vi "test-telemetry_engine.vi"() -> ()   [LabVIEW 2017, in "labview-standard-library.lvlib" / "data-logging.lvlib"]
uses:
  data-logging.lvlib
  <vilib>/Rock Robotics/WPI/DriverStation/WPI_DriverStationRobotMode2.ctl
panel:
  in  "Post dissable record time":dbl=10.0 format="%#_13g"
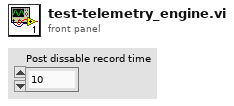
[diagram p1: front panel]
types:
  T1 = typedef "WPI_DriverStationRobotMode2.ctl" = enum16{"Autonomous Disabled", "Autonomous Enabled", "Teleop Disabled", "Teleop Enabled", "Disconnected", "Finish", "Test Disabled", "Test Enabled", "Emergency Stopped"}
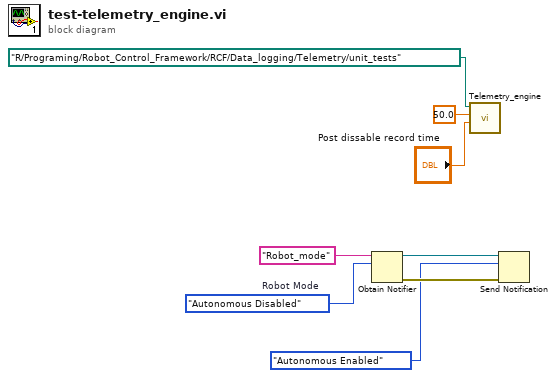
[diagram p0: block diagram]
diagram:
  w5 = WPI_DriverStationRobotMode2."Autonomous Disabled"  # Robot Mode
  n1 = Obtain Notifier(name (unnamed)="Robot_mode", notification data type=w5) -> (notifier out=w3:refnum<notifier>, error out=w2:errorcluster)  [unwired: 2 in, 1 out]
  n2 = call "Telemetry_engine.vi"("Post dissable record time"="Post dissable record time", "Recording rate (Hz)"=50.0, "Telemetry data folder path"=path "R:/Programing/Robot_Control_Framework/RCF/Data_logging/Telemetry/unit_tests") -> ()  [unwired: 9 in]
  n3 = Send Notification(notification=WPI_DriverStationRobotMode2."Autonomous Enabled", notifier=w3, error in (no error)=w2) -> ()  [unwired: 2 out]
